vi "XIPIN_Multiply_Adder_2_0.vi"   [LabVIEW 2017]
doc: "The Xilinx LogiCORE Multiply Adder generates a multiply-add function implemented in Xtreme DSP(TM) slices. User options allow you to specify the wordlengths of the inputs and output. Optimal pipelining for maximum speed and no pipelining are available.\n------------------------------------\n<b>Need License</b> : No"
uses:
  <vilib>/rvi/XilinxIP/XIPIN_XNode/niFpgaXIPIN.xnode
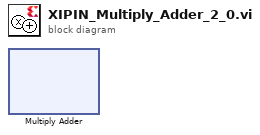
[diagram p0: block diagram]
diagram:
  n1 = xnode ("Multiply Adder")() -> ()
